vi "API POST Multipart File Upload.vi"(7 "Body Parameters Names":string[](array[string])=["id"], 8 "error in (no error)":errorcluster, 9 "FIlepath":path=path "D:/upwork/Labview-REST-API/labview-source/payload.png", 10 "API Token":string="apitoken 475eef11-95b9-4f32-9221-3162004815ef:f20a91a0-c04e-4d32-b0b4-337e6e91bde7", 11 "API Endpoint Url":string="https://api.dev.enlil.io/api/v1/attachments/external/upload") -> (0 "error out":errorcluster, 4 "Responce body":string, 5 "Responce headers":string, 6 "Body Parameters out":T1[](array[typedef]))   [LabVIEW 2017]
uses:
  Types/Body Parameter Type.ctl
  <vilib>/httpClient/MultipartData.ctl
  <vilib>/httpClient/LabVIEWHTTPClient.lvlib
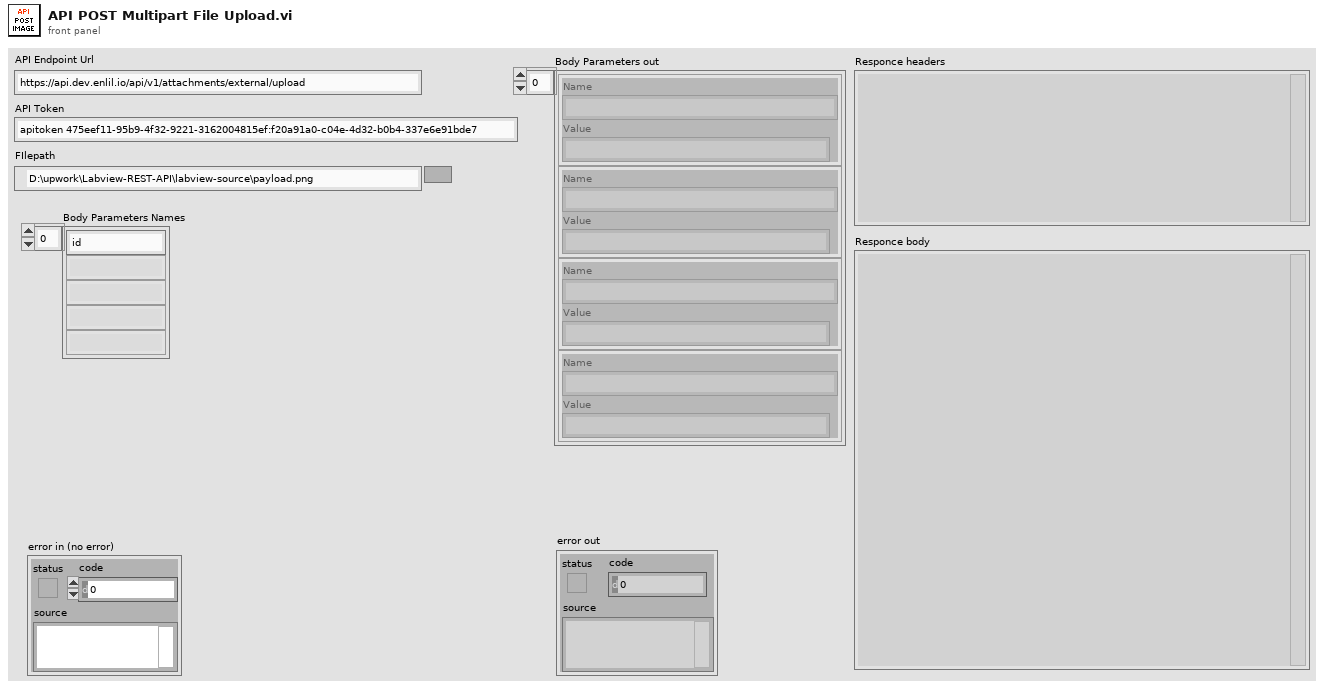
[diagram p1: front panel]
types:
  T1 = typedef "Body Parameter Type.ctl" = cluster{"Name":string, "Value":string}
  T2 = typedef "LabVIEWHTTPClient.lvlib/MultipartData.ctl" = cluster{"Name":string, "Value":string, "File":path, "Filename":string, "MIME type":string}
  T3 = typedef "LabVIEWHTTPClient.lvlib/ClientHandle.ctl" = refnum<k1>
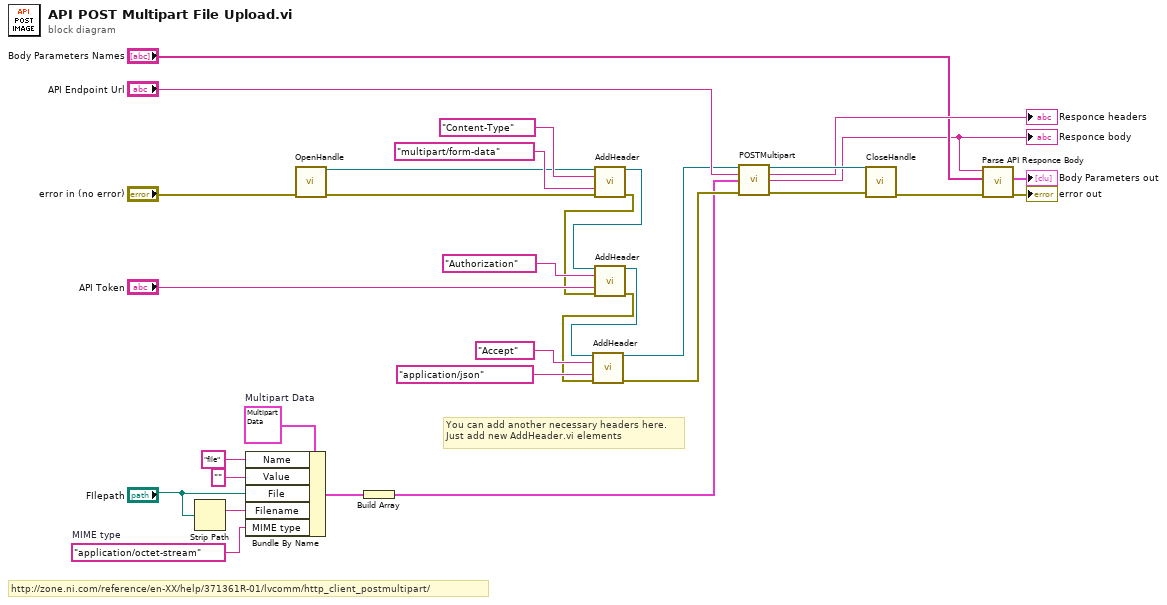
[diagram p0: block diagram]
diagram:
  w24 = "application/octet-stream"  # MIME type
  w28 = T2 {"Name"="", "Value"="", "File"=path "", "Filename"="", "MIME type"="application/octet-stream"}  # Multipart Data
  # "You can add another necessary headers here.\nJust add new AddHeader.vi elements"
  # "http://zone.ni.com/reference/en-XX/help/371361R-01/lvcomm/http_client_postmultipart/"
  n1 = Strip Path(path="FIlepath") -> (name=w25:string)  [unwired: 1 out]
  n2 = Bundle By Name(cluster=w28, "Name"="file", "Value"="", "File"="FIlepath", "Filename"=w25, "MIME type"=w24) -> (w23:T2)
  n3 = call <vilib>:"OpenHandle.vi"("error in (no error)"="error in (no error)") -> ("client handle out"=w11:T3, "error out"=w10:errorcluster)  [unwired: 13 in]
  n4 = Build Array(w23) -> (w7:T2[])
  n5 = call <vilib>:"AddHeader.vi"("client handle"=w11, "header"="Content-Type", "value"="multipart/form-data", "error in (no error)"=w10) -> ("client handle out"=w15:T3, "error out"=w14:errorcluster)  [unwired: 10 in]
  n6 = call <vilib>:"AddHeader.vi"("client handle"=w15, "header"="Authorization", "value"="API Token", "error in (no error)"=w14) -> ("client handle out"=w13:T3, "error out"=w12:errorcluster)  [unwired: 10 in]
  n7 = call <vilib>:"AddHeader.vi"("client handle"=w13, "header"="Accept", "value"="application/json", "error in (no error)"=w12) -> ("client handle out"=w9:T3, "error out"=w8:errorcluster)  [unwired: 10 in]
  n8 = call <vilib>:"POSTMultipart.vi"("client handle"=w9, "url"="API Endpoint Url", "data"=w7, "error in (no error)"=w8) -> ("client handle out"=w32:T3, "headers"=→"Responce headers":string, "body"=w2:string, "error out"=w31:errorcluster)  [unwired: 8 in]
  "Responce body" <- w2
  n9 = call <vilib>:"CloseHandle.vi"("client handle"=w32, "error in (no error)"=w31) -> ("error out"=w5:errorcluster)  [unwired: 13 in]
  n10 = call "Parse API Responce Body.vi"("error in (no error)"=w5, "Body Parameters Names in"="Body Parameters Names", "Response Body in"=w2) -> ("error out"=→"error out":errorcluster, "Body Parameters out"=→"Body Parameters out":T1[])  [unwired: 6 in, 1 out]
